vi "milliGAT_standalone_improvedStop.vi"() -> ()   [LabVIEW 2017]
uses:
  <vilib>/Instr/_visa.llb/VISA Configure Serial Port (Instr).vi
panel:
  in  "flow control":u16(ring) items=["None"=0, "XON/XOFF"=1, "RTS/CTS"=2, "DTR/DSR"=4]
  in  "stop bits":u16(ring)=10 items=["1.0"=10, "1.5"=15, "2.0"=20]
  in  "parity":u16(ring) items=["None", "Odd", "Even", "Mark", "Space"]
  in  "data bits":u16=8 min=5 max=8 step=1
  in  "VISA resource name":refnum<visa-resource-name>="COM1"
  in  "baud rate":u32=9600
  out "Answer":string
  in  "Tell":bool
  in  "?":u16(ring) items=["Constant flowrate, 0.0005<n<167uL/s", "Maximum flowrate, 0.001<n<167 uL/s", "Dispense Set Volume, 0.001<n<1E15 uL", "Aspirate Set Volume, 0.001<n<1E15 uL", "Stop Pump"]
  out "bytes read 2":u32
  in  "User Input":i32
  in  "Stop":bool
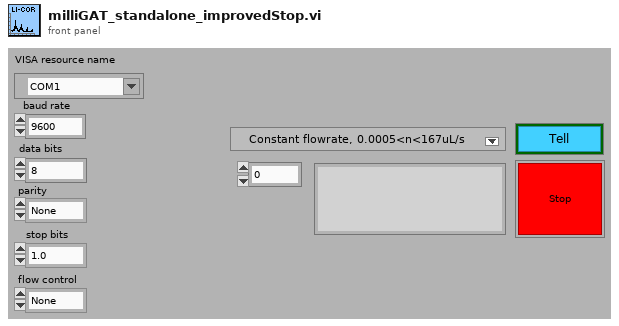
[diagram p1: front panel]
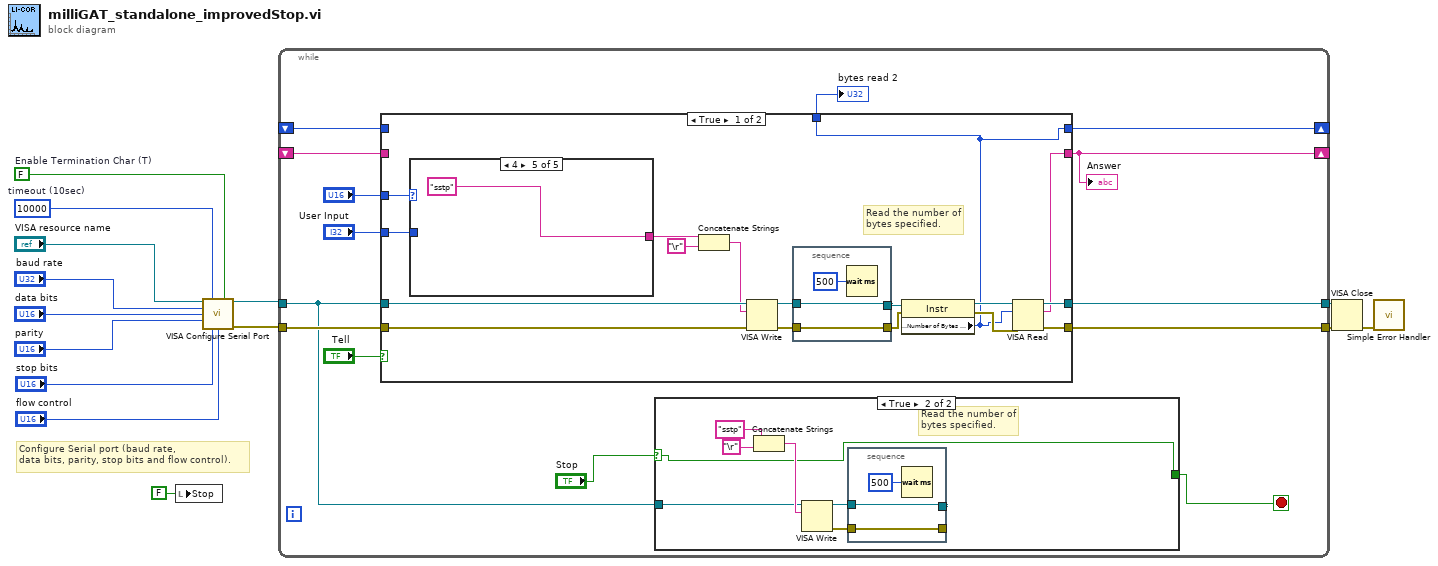
[diagram p0: block diagram]
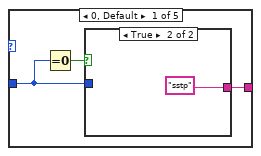
[diagram p3: hidden frame]
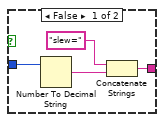
[diagram p4: hidden frame]
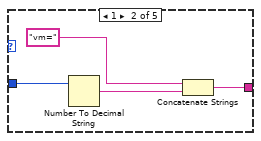
[diagram p5: hidden frame]
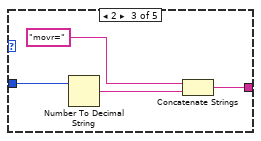
[diagram p6: hidden frame]
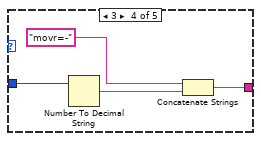
[diagram p7: hidden frame]
diagram:
  w7 = FALSE  # Enable Termination Char (T)
  w8 = u32 10000  # timeout (10sec)
  # "Configure Serial port (baud rate,\ndata bits, parity, stop bits and flow control)."
  n1 = local write "Stop"(FALSE ("Stop")) -> ()
  n2 = call-poly "VISA Configure Serial Port"("VISA resource name"="VISA resource name", "timeout (10sec)"=w8, "Enable Termination\nChar (T)"=w7, "baud rate (9600)"="baud rate", "data bits (8)"="data bits", "parity (0:none)"="parity", "stop bits (10: 1 bit)"="stop bits", "flow control (0:none)"="flow control") -> ("VISA resource name out"=w3:refnum<visa-resource-name>, "error out"=w2:errorcluster)  [unwired: 6 in]
  n3 = while {
    tunnel: w3 -> [w15]
    tunnel: w2 -> [w27]
    tunnel: [w25] -> w13
    tunnel: [w24] -> w12
    shift-right: [w21] -> _
    shift-left: _ -> [w20]
    shift-right: [w19] -> _
    shift-left: _ -> [w18]
    stop <- w16 stop-if-true
    n4 = case shown="True" "Tell" {
      tunnel: w15 -> [w49 w82]
      tunnel: w27 -> [w48 w81]
      tunnel: [w46 w82] -> w25
      tunnel: [w45 w81] -> w24
      tunnel: [w41 w83] -> w26
      tunnel: "User Input" -> [w44 _]
      tunnel: "?" -> [w42 _]
      tunnel: [w40 w84] -> w21
      tunnel: w20 -> [_ w84]
      tunnel: [w41 w83] -> w19
      tunnel: w18 -> [_ w83]
      frame True {
        # "Read the number of bytes specified."
        n5 = case shown="4" w42 {
          tunnel: [w59 w68 w72 w76 "sstp"] -> w56
          tunnel: w44 -> [w57 w67 w71 w75 _]
          frame 0, Default {
            n6 = Equal To 0?(x=w57) -> (x = 0?=w58:bool)
            n7 = case shown="True" w58 {
              tunnel: [w63 "sstp"] -> w59
              tunnel: w57 -> [w62 _]
              frame False {
                n8 = Number To Decimal String(number=w62) -> (decimal integer string=w60:string)  [unwired: 1 in]
                n9 = Concatenate Strings("slew=", w60) -> (w63:string)
              }
              frame True {
              }
            }
          }
          frame 1 {
            n10 = Number To Decimal String(number=w67) -> (decimal integer string=w65:string)  [unwired: 1 in]
            n11 = Concatenate Strings("vm=", w65) -> (w68:string)
          }
          frame 2 {
            n12 = Number To Decimal String(number=w71) -> (decimal integer string=w69:string)  [unwired: 1 in]
            n13 = Concatenate Strings("movr=", w69) -> (w72:string)
          }
          frame 3 {
            n14 = Number To Decimal String(number=w75) -> (decimal integer string=w73:string)  [unwired: 1 in]
            n15 = Concatenate Strings("movr=-", w73) -> (w76:string)
          }
          frame 4 {
          }
        }
        n16 = Concatenate Strings(w56, "\r") -> (w47:string)
        n17 = VISA Write(VISA resource name=w49, write buffer=w47, error in (no error)=w48) -> (VISA resource name out=w55:refnum<visa-resource-name>, error out=w54:errorcluster)  [unwired: 1 out]
        n18 = stacked-sequence {
          tunnel: w55 -> [w80]
          tunnel: w54 -> [w79]
          tunnel: [w80] -> w51
          tunnel: [w79] -> w50
          frame #0 {
            n19 = Wait (ms)(milliseconds to wait=u32 500) -> ()  [unwired: 1 out]
          }
        }
        n20 = property class="Instr"(reference=w51, error in=w50) -> (reference out=w53:refnum<visa-resource-name>, error out=w52:errorcluster, "Serial Settings:Number of Bytes at Serial Port"=w41:u32)
        n21 = VISA Read(VISA resource name=w53, byte count=w41, error in (no error)=w52) -> (VISA resource name out=w46:refnum<visa-resource-name>, read buffer=w40:string, error out=w45:errorcluster)  [unwired: 1 out]
      }
      frame False {
      }
    }
    "bytes read 2" <- w26
    "Answer" <- w21
    n22 = case shown="True" "Stop" {
      selector: "Stop" -> [w29 w31]
      tunnel: [w29 w31] -> w16
      tunnel: w15 -> [_ w30]
      frame False {
      }
      frame True {
        # "Read the number of bytes specified."
        n23 = Concatenate Strings("sstp" ("string"), "\r") -> (w34:string)
        n24 = VISA Write(VISA resource name=w30, write buffer=w34) -> (VISA resource name out=w36:refnum<visa-resource-name>, error out=w35:errorcluster)  [unwired: 1 in, 1 out]
        n25 = stacked-sequence {
          tunnel: w36 -> [w39]
          tunnel: w35 -> [w38]
          tunnel: [w39] -> _
          tunnel: [w38] -> _
          frame #0 {
            n26 = Wait (ms)(milliseconds to wait=u32 500) -> ()  [unwired: 1 out]
          }
        }
      }
    }
  }
  n27 = VISA Close(VISA resource name=w13, error in (no error)=w12) -> (error out=w14:errorcluster)
  n28 = call <vilib>:"Simple Error Handler.vi"("error in (no error)"=w14) -> ()  [unwired: 1 in, 8 out]
